vi "XYZStage-Move command.vi"(8 "Error In":errorcluster, 9 "XYZ Stage data":T1={"Command"=enum."Initialize", "Channel"="Z", "X"=0.0, "Y"=0.0, "Z"=0.0, "Speed"=0, "Zero"=FALSE, "Use acknowledgement?"=TRUE} {"Speed" format="Speed= %.0f"; "Z" format="Z= %#_g"; "Y" format="Y= %#_g"; "X" format="X= %#_g"}, 11 "XYZ Stage config":T4={"COM port"="COM7", "XY stage available"=FALSE}) -> (0 "Error Out":errorcluster, 1 "Move XYZ command String":string)   [LabVIEW 2013]
uses:
  Typedefs/XY Stage config cluster.ctl
  Typedefs/XYZ stage data.ctl
  Typedefs/XYZ stage states.ctl
  Typedefs/XYZ channel ring.ctl
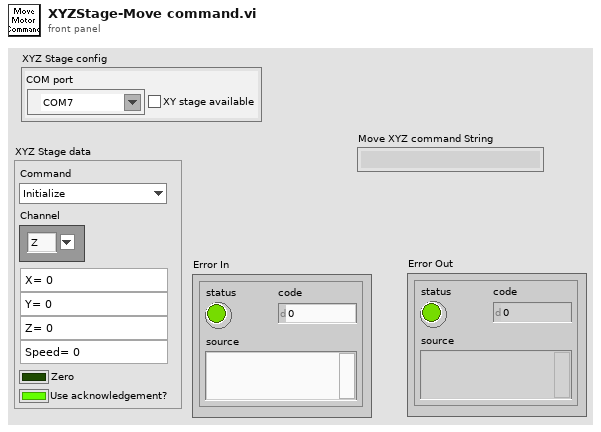
[diagram p1: front panel]
types:
  T1 = typedef "XYZ stage data.ctl" = cluster{"Command":T2, "Channel":T3, "X":sgl, "Y":sgl, "Z":sgl, "Speed":i32, "Zero":bool, "Use acknowledgement?":bool}
  T2 = typedef "XYZ stage states.ctl" = enum16{"Dequeue", "Initialize", "Read Position", "Read Speed Setting", "Move", "Set Max Speed", "Reset Axis", "Stop all movement"}
  T3 = typedef "XYZ channel ring.ctl" = string
  T4 = typedef "XY Stage config cluster.ctl" = cluster{"COM port":refnum<visa-resource-name>, "XY stage available":bool}
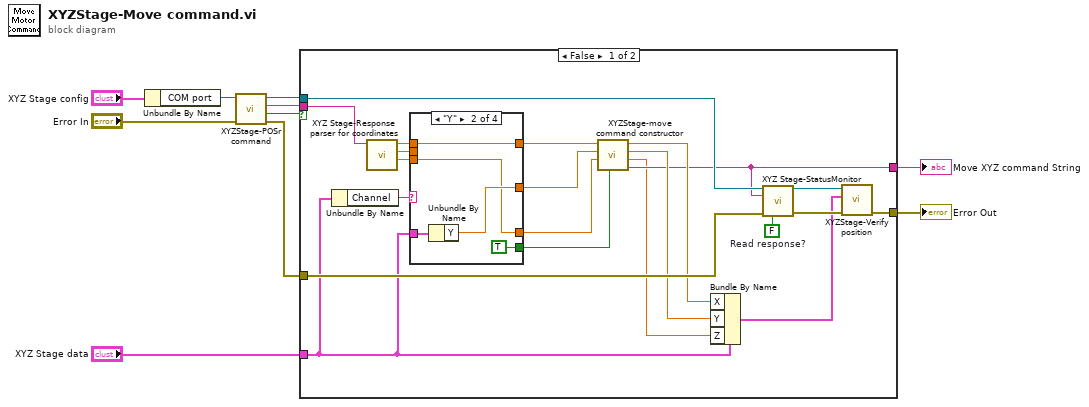
[diagram p0: block diagram]
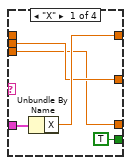
[diagram p2: hidden frame]
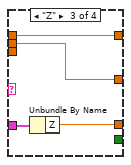
[diagram p3: hidden frame]
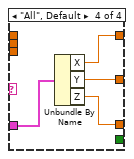
[diagram p4: hidden frame]
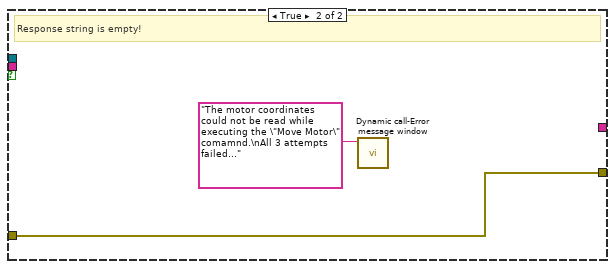
[diagram p5: hidden frame]
diagram:
  n1 = Unbundle By Name("XYZ Stage config") -> ("COM port"=w10:refnum<visa-resource-name>)
  n2 = call "XYZStage-POSr command.vi"("Error in"="Error In", "VISA Refnum in"=w10) -> ("Error out"=w1:errorcluster, "Empty response string"=w3:bool, "read string"=w9:string, "VISA Refnum out"=w7:refnum<visa-resource-name>)  [unwired: 6 in]
  n3 = case shown="False" w3 {
    tunnel: w1 -> [w31 w51]
    tunnel: w9 -> [w30 _]
    tunnel: w7 -> [w29 _]
    tunnel: [w23 w51] -> w6
    tunnel: "XYZ Stage data" -> [w19 _]
    tunnel: [w15 _] -> w4
    frame False {
      w21 = FALSE  # Read response?
      n4 = Unbundle By Name(w19) -> ("Channel"=w28:T3)
      n5 = call "XYZ Stage-Response parser for coordinates.vi"("Filtered response string (no CR)"=w30) -> ("Z"=w25:sgl, "Y"=w26:sgl, "X"=w27:sgl)  [unwired: 8 in]
      n6 = case shown="\"Y\"" w28 {
        tunnel: [w35 w40 w43 w49] -> w14
        tunnel: [w34 w39 w42 w48] -> w20
        tunnel: [w33 w38 w44 w47] -> w13
        tunnel: w19 -> [w36 w41 w45 w46]
        tunnel: w27 -> [_ w40 w43 _]
        tunnel: w26 -> [w34 _ w42 _]
        tunnel: w25 -> [w33 w38 _ _]
        tunnel: [TRUE TRUE _ _] -> w11
        frame "X" {
          n7 = Unbundle By Name(w36) -> ("X"=w35:sgl)
        }
        frame "Y" {
          n8 = Unbundle By Name(w41) -> ("Y"=w39:sgl)
        }
        frame "Z" {
          n9 = Unbundle By Name(w45) -> ("Z"=w44:sgl)
        }
        frame "All", Default {
          n10 = Unbundle By Name(w46) -> ("X"=w49:sgl, "Y"=w48:sgl, "Z"=w47:sgl)
        }
      }
      n11 = call "XYZStage-move command constructor.vi"("Bypass Z-safety interlock"=w11, "Z"=w13, "Y"=w20, "X"=w14) -> ("Move command"=w15:string, "Adjusted Z"=w12:sgl, "Adjusted Y"=w16:sgl, "Adjusted X"=w17:sgl)  [unwired: 4 in]
      n12 = Bundle By Name(cluster=w19, "X"=w17, "Y"=w16, "Z"=w12) -> (w18:T1)
      n13 = call "XYZ Stage-StatusMonitor.vi"("VISA resource name"=w29, "string to write"=w15, "Error In"=w31, "Read response? (T)"=w21) -> ("VISA resource name out"=w22:refnum<visa-resource-name>, "Error Out"=w24:errorcluster)  [unwired: 7 in, 3 out]
      n14 = call "XYZStage-Verify position.vi"("error in (no error)"=w24, "XYZ Stage data"=w18, "XYZ Stage Port"=w22) -> ("error out"=w23:errorcluster)  [unwired: 8 in]
    }
    frame True {
      # "Response string is empty!"
      n15 = call "Dynamic call-Error message window.vi"("Error Message"="The motor coordinates could not be read while executing the \"Move Motor\" comamnd.\nAll 3 attempts failed...") -> ()  [unwired: 10 in, 1 out]
    }
  }
  "Move XYZ command String" <- w4
  "Error Out" <- w6
